vi "CallingVI.vi"() -> ()   [LabVIEW 2009]
uses:
  TimerCommands.ctl
panel:
  in  "Temps cible (s)":dbl
  out "Temps écoulé":dbl
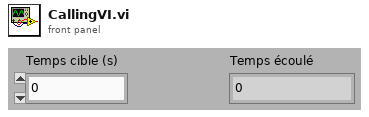
[diagram p1: front panel]
types:
  T1 = typedef "TimerCommands.ctl" = enum16{"Démarrer", "Vérifier le temps"}
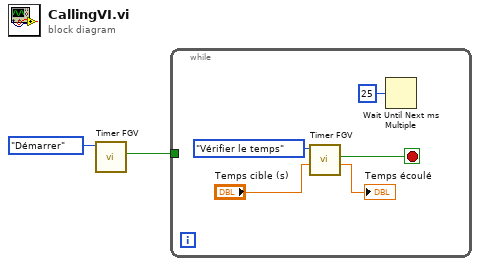
[diagram p0: block diagram]
diagram:
  n1 = call "Timer FGV.vi"("Commande du timer"=TimerCommands."Démarrer" ("Timer Command")) -> ("Terminé ?"=w2:bool)  [unwired: 9 in, 1 out]
  n2 = while "Boucle While" {
    tunnel: w2 -> [_]
    stop <- w6 stop-if-true
    n3 = call "Timer FGV.vi"("Temps cible (s)"="Temps cible (s)", "Commande du timer"=TimerCommands."Vérifier le temps" ("Timer Command")) -> ("Temps écoulé"=→"Temps écoulé":dbl, "Terminé ?"=w6:bool)  [unwired: 8 in]
    n4 = Wait Until Next ms Multiple ("Attendre un multiple de ms")(millisecond multiple=u32 25) -> ()  [unwired: 1 out]
  }
